vi "LJLogM write to file.vi"(0 "Data File Reference In":path, 1 "Is Log Interval?":bool, 2 "Data File Prefix":string, 5 "Working Directory":path, 7 "Timestamp":timestamp, 9 "Channel Names":string[](array[string]), 11 "Channel Data":dbl[](array[numeric]), 12 "Max File Size (Bytes)":i32, 13 "Write to file?":bool) -> (4 "Data File Reference Out":path, 6 "Working Directory Out":path)   [LabVIEW 2026]
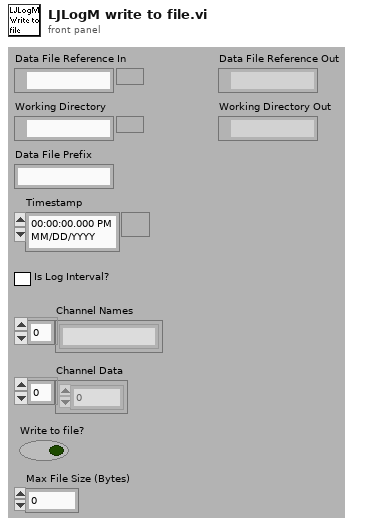
[diagram p1: front panel]
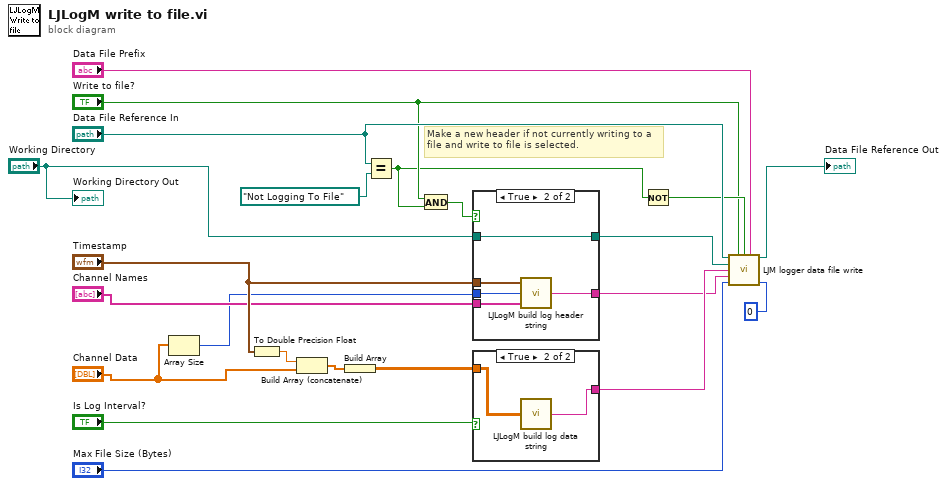
[diagram p0: block diagram]
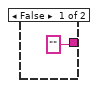
[diagram p2: hidden frame]
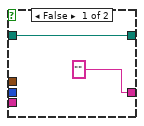
[diagram p3: hidden frame]
diagram:
  # "Make a new header if not currently writing to a file and write to file is selected."
  n1 = Array Size(array="Channel Data") -> (size(s)=w14:i32)
  n2 = To Double Precision Float(number="Timestamp") -> (double precision float=w5:dbl)
  n3 = Build Array (concatenate)(w5, "Channel Data") -> (w8:dbl[])
  n4 = Build Array(w8) -> (w7:dbl[][])
  n5 = Equal?(x="Data File Reference In", y=path "Not Logging To File") -> (x = y?=w3:bool)
  n6 = And(x="Write to file?", y=w3) -> (x .and. y?=w1:bool)
  n7 = case shown="True" w1 {
    tunnel: w14 -> [_ w29]
    tunnel: "Channel Names" -> [_ w28]
    tunnel: ["" ("Header String") w27] -> w11
    tunnel: "Working Directory" -> [w23 w26]
    tunnel: [w23 w26] -> w10
    tunnel: "Timestamp" -> [_ w25]
    frame False {
    }
    frame True {
      n8 = call "LJLogM build log header string.vi"("Names"=w28, "# Channels"=w29, "Start Timestamp"=w25) -> ("Header String"=w27:string)
    }
  }
  n9 = case shown="True" "Is Log Interval?" {
    tunnel: ["" ("Output data") w32] -> w12
    tunnel: w7 -> [_ w31]
    frame False {
    }
    frame True {
      n10 = call "LJLogM build log data string.vi"("Data"=w31) -> ("Output data"=w32:string)
    }
  }
  n11 = Not(x=w3) -> (.not. x?=w9:bool)
  n12 = call "LJM logger data file write.vi"("Current Data File In"="Data File Reference In", "Write To File"="Write to file?", "Currently Writing"=w9, "Data File Prefix"="Data File Prefix", "Working Directory"=w10, "Log data"=w12, "Header String"=w11, "max file size (bytes)"="Max File Size (Bytes)", "Starting #"=u32 0 ("Data File #")) -> ("Current Data File Out"=→"Data File Reference Out":path)  [unwired: 5 in, 1 out]
  "Working Directory Out" <- "Working Directory"
